vi "dfd_Convert String to Multirate Filter.vi"(8 "error in (no error)":errorcluster, 10 "xml string":string, 11 "multirate filter in":T1={"mMRate_Structure"=enum."IIR", "mMRate_Mode"=0, "mMRate_Factor"=-1, "mMRate_FIRParams"={"mMRate_FIR_H"=[], "mMRate_FIR_IsNyquist?"=FALSE, "mMRate_FIR_IsSymmetric?"=FALSE}, "mMRate_CICParams"={"mMRate_CIC_#Stage"=0, "mMRate_CIC_Lag"=0, "mMRate_CIC_Type"=enum."Lowpass"}, "mMRate_Order"=0, "mMRate_Version"="2.0", "mMRate_Comments"="", "mMRate_RationalFactor"={"mMRate_L"=-1, "mMRate_M"=-1}, "mMRate_Fs"=1.0, "mMRate_Quantized?"=FALSE, "mMRate_QFilterGain"=1.0, "mMRate_CoefWl"=16, "mMRate_Scaling"={"mMRate_ScaleByPowerOf2?"=FALSE, "mMRate_ScaleType"=enum."No Norm"}, "mMRate_InputWl"=16, "mMRate_OutputWl"=16, "mMRate_OutputMode"=enum."Truncation", "mMRate_MultMode"=enum."Truncated", "mMRate_BitPruning"=FALSE, "mMRate_GainWl"=16, "mMRate_OutputFwl"=0, "mMRate_SumIwl"=0, "mMRate_InputIwl "=16, "mMRate_SumWl"=32, "mMRate_CoefIwl"=0} {"mMRate_SumWl" min=1 max=32 step=1; "mMRate_InputIwl" min=1 max=32 step=1; "mMRate_GainWl" min=1 max=32 step=1; "mMRate_OutputWl" min=1 max=32 step=1; "mMRate_InputWl" min=1 max=32 step=1; "mMRate_CoefWl" min=1 max=32 step=1; "mMRate_Mode" items=["Default"=-1, "No Rate Change"=0, "Interpolation"=1, "Decimation"=2, "Interpolated"=3, "Rational"=4]}) -> (0 "error out":errorcluster, 3 "multirate filter out":T1={"mMRate_Structure"=enum."IIR", "mMRate_Mode"=0, "mMRate_Factor"=-1, "mMRate_FIRParams"={"mMRate_FIR_H"=[], "mMRate_FIR_IsNyquist?"=FALSE, "mMRate_FIR_IsSymmetric?"=FALSE}, "mMRate_CICParams"={"mMRate_CIC_#Stage"=0, "mMRate_CIC_Lag"=0, "mMRate_CIC_Type"=enum."Lowpass"}, "mMRate_Order"=0, "mMRate_Version"="2.0", "mMRate_Comments"="", "mMRate_RationalFactor"={"mMRate_L"=-1, "mMRate_M"=-1}, "mMRate_Fs"=1.0, "mMRate_Quantized?"=FALSE, "mMRate_QFilterGain"=1.0, "mMRate_CoefWl"=16, "mMRate_Scaling"={"mMRate_ScaleByPowerOf2?"=FALSE, "mMRate_ScaleType"=enum."No Norm"}, "mMRate_InputWl"=16, "mMRate_OutputWl"=16, "mMRate_OutputMode"=enum."Truncation", "mMRate_MultMode"=enum."Truncated", "mMRate_BitPruning"=FALSE, "mMRate_GainWl"=16, "mMRate_OutputFwl"=0, "mMRate_SumIwl"=0, "mMRate_InputIwl "=16, "mMRate_SumWl"=32, "mMRate_CoefIwl"=0} {"mMRate_SumWl" min=1 max=32 step=1; "mMRate_InputIwl" min=1 max=32 step=1; "mMRate_GainWl" min=1 max=32 step=1; "mMRate_OutputWl" min=1 max=32 step=1; "mMRate_InputWl" min=1 max=32 step=1; "mMRate_CoefWl" min=1 max=32 step=1; "mMRate_Mode" items=["Default"=-1, "No Rate Change"=0, "Interpolation"=1, "Decimation"=2, "Interpolated"=3, "Rational"=4]})   [LabVIEW 2017, in "NI_DigFilter_Process.lvlib"]
uses:
  <vilib>/addons/Digital Filter Design/NI_DigFilter_Process.lvlib
  <vilib>/addons/Digital Filter Design/_Objects.llb/DFD Multirate Filter Obj.ctl
  <vilib>/addons/Digital Filter Design/_Objects.llb/DFD Multirate Mode.ctl
  <vilib>/addons/Digital Filter Design/_Objects.llb/DFD Coef Norm Type.ctl
  <vilib>/addons/Digital Filter Design/_Objects.llb/DFD Round-off Mode.ctl
  <vilib>/addons/Digital Filter Design/_Objects.llb/DFD FXP MRate Multiply Mode.ctl
  <vilib>/addons/Digital Filter Design/NI_DigFilterLicensed.lvlib
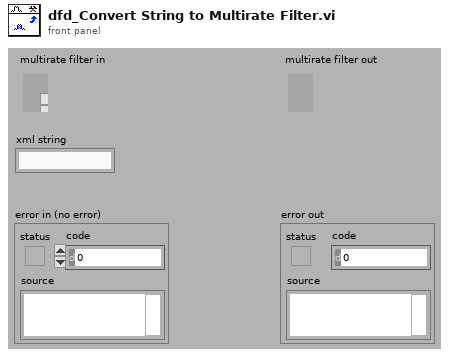
[diagram p1: front panel]
types:
  T1 = typedef "NI_DigFilterLicensed.lvlib/DFD Multirate Filter Obj.ctl" = cluster{"mMRate_Structure":enum16{"CIC", "FIR", "IIR", "Lattice"}, "mMRate_Mode":T2, "mMRate_Factor":i32, "mMRate_FIRParams":cluster{"mMRate_FIR_H":dbl[], "mMRate_FIR_IsNyquist?":bool, "mMRate_FIR_IsSymmetric?":bool}, "mMRate_CICParams":cluster{"mMRate_CIC_#Stage":i32, "mMRate_CIC_Lag":i32, "mMRate_CIC_Type":enum16{"Lowpass", "Highpass"}}, "mMRate_Order":i32, "mMRate_Version":string, "mMRate_Comments":string, "mMRate_RationalFactor":cluster{"mMRate_L":i32, "mMRate_M":i32}, "mMRate_Fs":dbl, "mMRate_Quantized?":bool, "mMRate_QFilterGain":dbl, "mMRate_CoefWl":i16, "mMRate_Scaling":cluster{"mMRate_ScaleByPowerOf2?":bool, "mMRate_ScaleType":T3}, "mMRate_InputWl":i16, "mMRate_OutputWl":i16, "mMRate_OutputMode":T4, "mMRate_MultMode":T5, "mMRate_BitPruning":bool, "mMRate_GainWl":i16, "mMRate_OutputFwl":i16, "mMRate_SumIwl":i16, "mMRate_InputIwl ":i16, "mMRate_SumWl":i16, "mMRate_CoefIwl":i16}
  T2 = typedef "NI_DigFilterLicensed.lvlib/DFD Multirate Mode.ctl" = i16
  T3 = typedef "NI_DigFilterLicensed.lvlib/DFD Coef Norm Type.ctl" = enum16{"No Norm", "Time Domain 1-Norm", "Time Domain 2-Norm", "Time Domain Inf-Norm"}
  T4 = typedef "NI_DigFilterLicensed.lvlib/DFD Round-off Mode.ctl" = enum16{"Nearest", "Truncation"}
  T5 = typedef "NI_DigFilterLicensed.lvlib/DFD FXP MRate Multiply Mode.ctl" = enum16{"Truncated", "Full"}
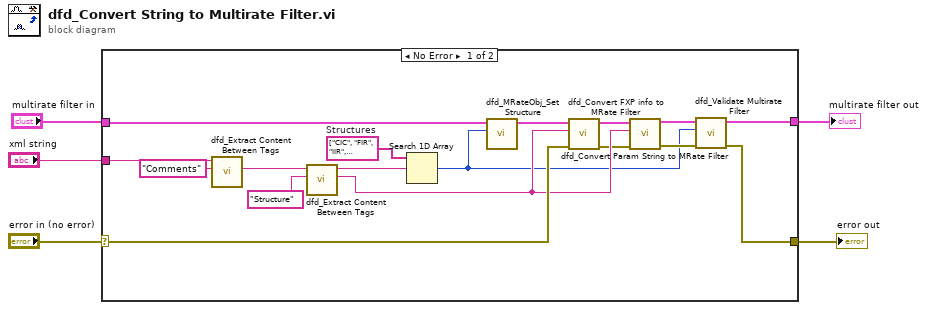
[diagram p0: block diagram]
diagram:
  n1 = case shown="No Error" "error in (no error)" {
    selector: "error in (no error)" -> [w15 w24]
    tunnel: "xml string" -> [w22 _]
    tunnel: "multirate filter in" -> [w17 w23]
    tunnel: [w9 w23] -> w1
    tunnel: [w11 w24] -> w4
    frame No Error {
      w6 = string[] ["CIC", "FIR", "IIR", "Lattice"]  # Structures
      n2 = call <vilib>:"dfd_Extract Content Between Tags.vi"("element"="Comments", "xml string with tag"=w22) -> ("remaining string"=w19:string)  [unwired: 9 out]
      n3 = call <vilib>:"dfd_Extract Content Between Tags.vi"("element"="Structure", "xml string with tag"=w19) -> ("remaining string"=w13:string, "content"=w18:string)  [unwired: 8 out]
      n4 = Search 1D Array(1D array=w6, element=w18) -> (index of element=w8:i32)  [unwired: 1 out]
      n5 = call <vilib>:"dfd_MRateObj_Set Structure.vi"("structure"=w8, "multirate filter in"=w17) -> ("multirate filter out"=w16:T1)  [unwired: 1 in, 8 out]
      n6 = call <vilib>:"dfd_Convert FXP info to MRate Filter.vi"("error in (no error)"=w15, "xml string in"=w13, "multirate filter in"=w16) -> ("error out"=w12:errorcluster, "multirate filter out"=w14:T1)  [unwired: 7 out]
      n7 = call <vilib>:"dfd_Convert Param String to MRate Filter.vi"("error in (no error)"=w12, "xml string in"=w13, "multirate filter in"=w14) -> ("error out"=w10:errorcluster, "dup multirate filter"=w7:T1)  [unwired: 7 out]
      n8 = call <vilib>:"dfd_Validate Multirate Filter.vi"("error in (no error)"=w10, "preferred structure"=w8, "multirate filter in"=w7) -> ("error out"=w11:errorcluster, "multirate filter out"=w9:T1)  [unwired: 1 in, 6 out]
    }
    frame Error {
    }
  }
  "error out" <- w4
  "multirate filter out" <- w1
